vi "Up Down Hall.vi"() -> ()   [LabVIEW 2025]
uses:
  6c21c491-3613-49b9-8739-58848ace7e6b.vi
  9d677228-37d7-4fae-91d8-cc659d765936.vi
  9a2c7101-15d1-4822-83f9-fc476c468639.vi
  af5d74b8-55dd-445e-b05f-4c49f1f30415.vi
panel:
  in  "Save Path":path
  in  "Stop":bool
  in  "Save":bool
  in  "Configuration":T1={"Up file"=path "\\\\myhome\\NHMFLDATA/Data/Cell8daq/Mijkhail Eremets_P20272-E005-PF/October_2025/100825/p154355_100825.tdms", "Down file"=path "\\\\myhome\\NHMFLDATA/Data/Cell8daq/Mijkhail Eremets_P20272-E005-PF/October_2025/100825/p171857_100825.tdms", "Invert X"=TRUE, "Bin data"=enum."Down", "Bin size"=0.1, "Chan Vxy X"="V X1 (Resampled)", "Chan Vxy Y"="V Y1 (Resampled)", "Chan X"="Field (Resampled)", "Group"="p", "Phase"=20.31092436974791, "Delta Phase"=-1.3313253012048292, "Averaging"=0.0, "Output file name"="Hall_250K", "VHall Volts to Ohms"=7.7, "Reference Rhall"=0.0, "Save with zero offset"=TRUE} {"Delta Phase" step=0.05 scale=-180.0..180.0; "Phase" scale=-180.0..180.0}
  out "Hall":T2(graph)
  out "Vxy":T2(graph)
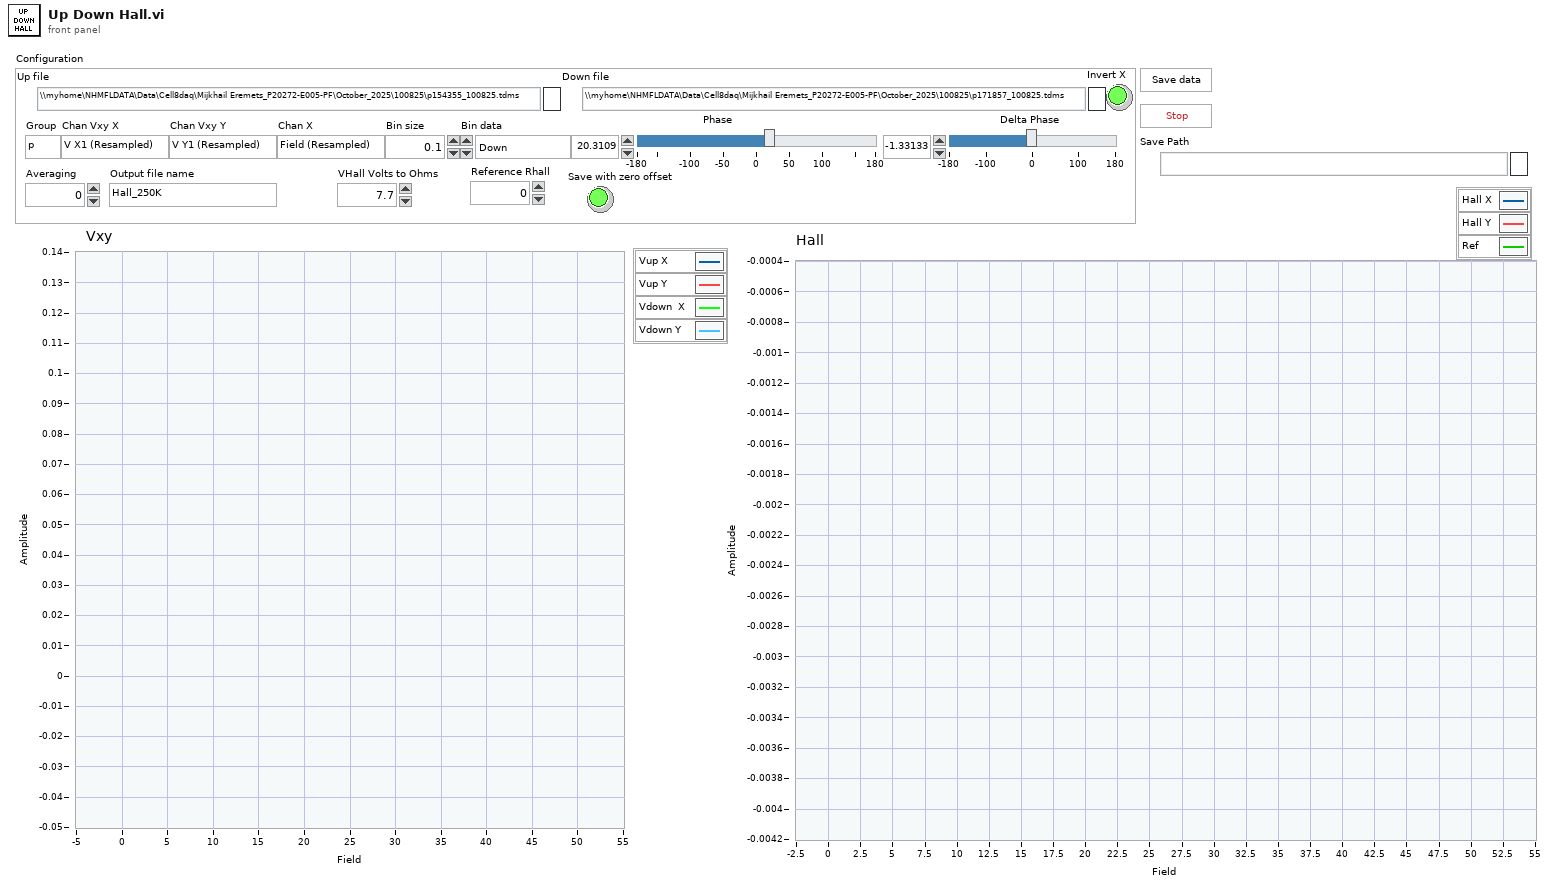
[diagram p1: front panel]
types:
  T1 = cluster{"Up file":path, "Down file":path, "Invert X":bool, "Bin data":enum16{"NONE", "Up", "Down", "Up+Down"}, "Bin size":dbl, "Chan Vxy X":string, "Chan Vxy Y":string, "Chan X":string, "Group":string, "Phase":dbl, "Delta Phase":dbl, "Averaging":dbl, "Output file name":string, "VHall Volts to Ohms":dbl, "Reference Rhall":dbl, "Save with zero offset":bool}
  T2 = cluster{"Binned data up":dbl[], "Binned data up":dbl[]}[]
  T3 = enum16{"open", "open or create", "create or replace", "create", "open (read-only)"}
  T4 = cluster{"Binned data down":dbl[], "Array X out":dbl[]}
  T5 = cluster{"Binned data down":dbl[], "Array Y out":dbl[]}
  T6 = cluster{"Binned data down":dbl[], "Array Y out":dbl[]}[]
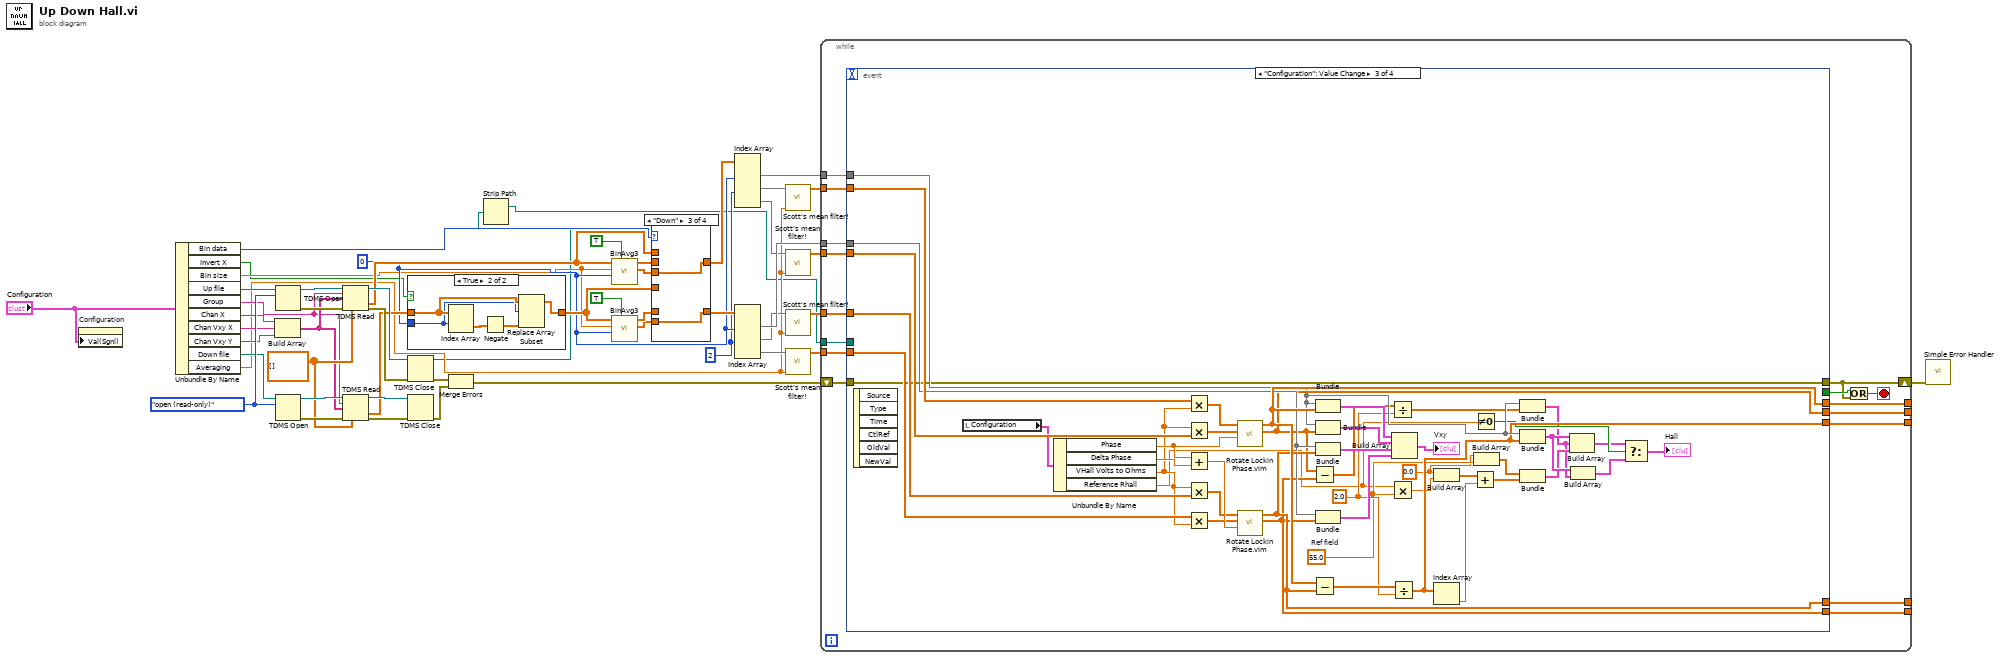
[diagram p0: block diagram]
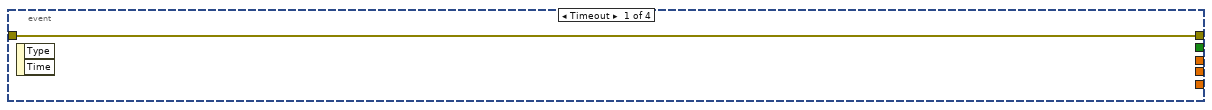
[diagram p3: hidden frame]
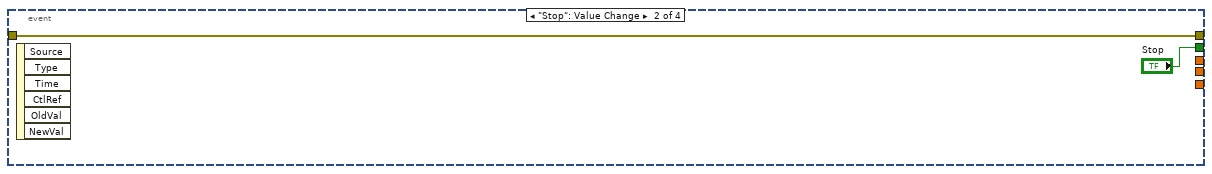
[diagram p4: hidden frame]
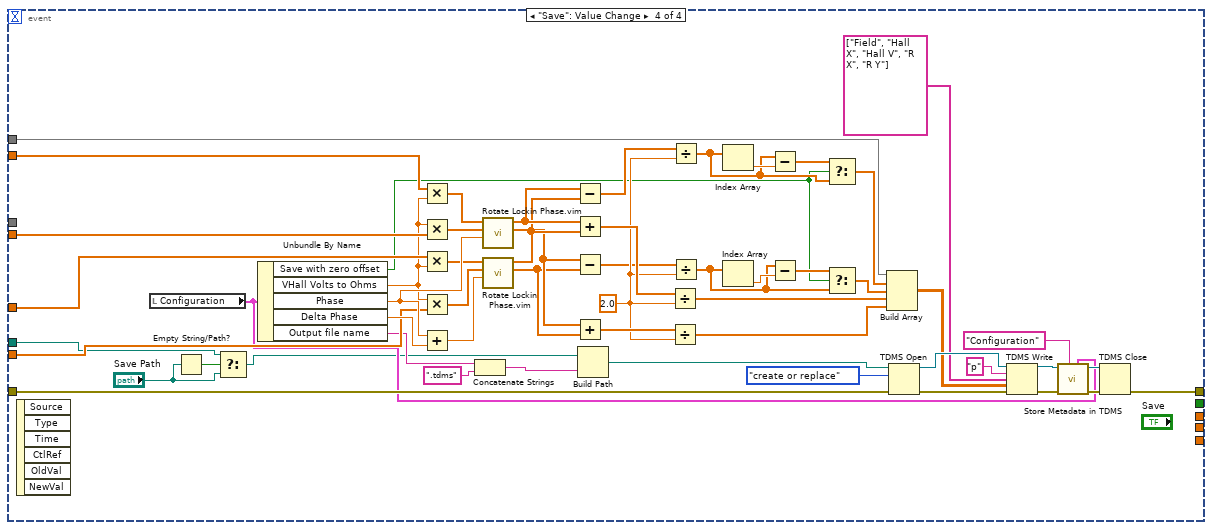
[diagram p5: hidden frame]
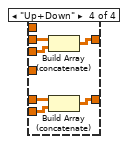
[diagram p8: hidden frame]
diagram:
  w20 = 2 ("index (row)")
  w21 = 0 ("index (row)")
  w42 = dbl[][] []
  w43 = T3."open (read-only)" ("operation (0:open)")
  n1 = property on="Configuration" class="Clust (strict)"("Val(Sgnl)"="Configuration") -> ()  [unwired: 2 in, 2 out]
  n2 = Unbundle By Name("Configuration") -> ("Bin data"=w8:enum16{"NONE", "Up", "Down", "Up+Down"}, "Invert X"=w7:bool, "Bin size"=w11:dbl, "Up file"=w19:path, "Group"=w15:string, "Chan X"=w16:string, "Chan Vxy X"=w18:string, "Chan Vxy Y"=w17:string, "Down file"=w14:path, "Averaging"=w10:dbl)
  n3 = Build Array(w16, w18, w17) -> (w41:string[])
  n4 = TDMS Open(10:w43, 11:w19) -> (0:w50:errorcluster, 3:w51:refnum<k34>)  [unwired: 5 in]
  n5 = TDMS Open(10:w43, 11:w14) -> (0:w45:errorcluster, 3:w44:refnum<k34>)  [unwired: 5 in]
  n6 = TDMS Read(0:w51, 5:w15, 7:w41, 11:w50, 12:w42) -> (4:w48:refnum<k34>, 10:w38:dbl[][], 15:w49:errorcluster)  [unwired: 3 in, 3 out]
  n7 = TDMS Read(0:w44, 5:w15, 7:w41, 11:w45, 12:w42) -> (4:w47:refnum<k34>, 10:w23:dbl[][], 15:w46:errorcluster)  [unwired: 3 in, 3 out]
  n8 = case shown="True" w7 {
    tunnel: w23 -> [w52 w57]
    tunnel: w21 -> [_ w54]
    tunnel: [w52 w53] -> w22
    frame False {
    }
    frame True {
      n9 = Index Array(array=w57, index (row)=w54) -> (element=w56:dbl[])  [unwired: 1 in]
      n10 = Negate(x=w56) -> (-x=w55:dbl[])
      n11 = Replace Array Subset(array=w57, new element=w55, index (row)=w54) -> (w53:dbl[][])  [unwired: 1 in]
    }
  }
  n12 = TDMS Close(8:w49, 11:w48) -> (0:w3:errorcluster, 3:w6:path)
  n13 = TDMS Close(8:w46, 11:w47) -> (0:w4:errorcluster)  [unwired: 1 out]
  n14 = Merge Errors(w3, w4) -> (w2:errorcluster)
  n15 = Strip Path(path=w6) -> (stripped path=w5:path)  [unwired: 1 out]
  n16 = call "BinAvg3.vi"("Extend to 0"=TRUE, "X coumn index"=w21, "Bin size"=w11, "Data in"=w38) -> ("Binned data down"=w36:dbl[][], "Binned data up"=w39:dbl[][])  [unwired: 6 in]
  n17 = call "BinAvg3.vi"("Extend to 0"=TRUE, "X coumn index"=w21, "Bin size"=w11, "Data in"=w22) -> ("Binned data down"=w37:dbl[][], "Binned data up"=w40:dbl[][])  [unwired: 6 in]
  n18 = case shown="\"Down\"" w8 {
    tunnel: w40 -> [_ w61 _ w69]
    tunnel: [w59 w61 w63 w67] -> w29
    tunnel: w39 -> [_ w60 _ w66]
    tunnel: [w58 w60 w62 w64] -> w35
    tunnel: w22 -> [w59 _ _ _]
    tunnel: w38 -> [w58 _ _ _]
    tunnel: w37 -> [_ _ w63 w68]
    tunnel: w36 -> [_ _ w62 w65]
    frame "NONE", Default {
    }
    frame "Up" {
    }
    frame "Down" {
    }
    frame "Up+Down" {
      n19 = Build Array (concatenate)(w66, w65) -> (w64:dbl[][])
      n20 = Build Array (concatenate)(w69, w68) -> (w67:dbl[][])
    }
  }
  n21 = Index Array(array=w35, index (col) #1=w21, index (col) #2=w20) -> (element #1=w34:dbl[], element #2=w25:dbl[], element #3=w24:dbl[])  [unwired: 4 in]
  n22 = Index Array(array=w29, index (col) #1=w21, index (col) #2=w20) -> (element #1=w28:dbl[], element #2=w27:dbl[], element #3=w26:dbl[])  [unwired: 4 in]
  n23 = call "Scott's mean filter!.vi"("window size"=w10, "input"=w25) -> ("output"=w33:dbl[])  [unwired: 9 out]
  n24 = call "Scott's mean filter!.vi"("window size"=w10, "input"=w24) -> ("output"=w32:dbl[])  [unwired: 9 out]
  n25 = call "Scott's mean filter!.vi"("window size"=w10, "input"=w27) -> ("output"=w31:dbl[])  [unwired: 9 out]
  n26 = call "Scott's mean filter!.vi"("window size"=w10, "input"=w26) -> ("output"=w30:dbl[])  [unwired: 9 out]
  n27 = while {
    tunnel: [w78] -> _
    tunnel: [w80] -> _
    tunnel: [w77] -> _
    tunnel: [w81] -> _
    tunnel: [w79] -> _
    tunnel: w30 -> [w82]
    tunnel: w31 -> [w83]
    tunnel: w32 -> [w84]
    tunnel: w33 -> [w85]
    tunnel: w34 -> [w75]
    tunnel: w28 -> [w74]
    tunnel: w5 -> [w73]
    shift-right: [w71] -> w1
    shift-left: w2 -> [w70]
    stop <- w72 stop-if-true
    n28 = event shown="[2] \"Configuration\": Value Change" {
      selector: _ -> [_ _ _ _]
      dyn-events: _ -> [_ _ _ _]
      timeout: _ -> [_ _ _ _]
      tunnel: w85 -> [_ _ w133 w184]
      tunnel: w84 -> [_ _ w132 w183]
      tunnel: w83 -> [_ _ w131 w151]
      tunnel: w82 -> [_ _ w130 w182]
      tunnel: [_ _ w121 _] -> w81
      tunnel: [_ _ w120 _] -> w80
      tunnel: [_ _ w129 _] -> w79
      tunnel: [_ _ w104 _] -> w78
      tunnel: [_ _ w125 _] -> w77
      tunnel: [_ "Stop" _ _] -> w76
      tunnel: w75 -> [_ _ w119 w185]
      tunnel: w74 -> [_ _ w124 _]
      tunnel: w73 -> [_ _ _ w148]
      tunnel: w70 -> [w86 w87 w114 w178]
      tunnel: [w86 w87 w114 w173] -> w71
      event Timeout {
        n29 = event-data() -> ()  [unwired: 3 out]
      }
      event "Stop": Value Change {
        n30 = event-data() -> ()  [unwired: 7 out]
      }
      event "Configuration": Value Change {
        w100 = 0.0 ("element")
        w101 = 55.0  # Ref field
        w105 = 2.0
        n31 = event-data() -> ()  [unwired: 7 out]
        n32 = local read "Configuration"() -> (w117:T1)
        n33 = Unbundle By Name(w117) -> ("Phase"=w116:dbl, "Delta Phase"=w115:dbl, "VHall Volts to Ohms"=w109:dbl, "Reference Rhall"=w90:dbl)
        n34 = Multiply(x=w133, y=w109) -> (x*y=w113:dbl[])
        n35 = Multiply(x=w109, y=w132) -> (x*y=w112:dbl[])
        n36 = Add(x=w116, y=w115) -> (x+y=w118:dbl)
        n37 = Multiply(x=w109, y=w131) -> (x*y=w111:dbl[])
        n38 = Multiply(x=w130, y=w109) -> (x*y=w110:dbl[])
        n39 = call "Rotate Lockin Phase.vim"("Phase"=w116, "Array Y in"=w112, "Array X in"=w113) -> ("Array Y out"=w121:dbl[], "Array X out"=w129:dbl[])  [unwired: 7 in]
        n40 = call "Rotate Lockin Phase.vim"("Phase"=w118, "Array Y in"=w110, "Array X in"=w111) -> ("Array Y out"=w120:dbl[], "Array X out"=w125:dbl[])  [unwired: 7 in]
        n41 = Subtract(x=w121, y=w120) -> (x-y=w107:dbl[])
        n42 = Subtract(x=w129, y=w125) -> (x-y=w106:dbl[])
        n43 = Bundle("Binned data down"=w119, "Array X out"=w129) -> (w128:T4)  [unwired: 1 in]
        n44 = Bundle("Binned data down"=w119, "Array Y out"=w121) -> (w127:T5)  [unwired: 1 in]
        n45 = Bundle("Binned data down"=w124, "Array X out"=w125) -> (w122:T4)  [unwired: 1 in]
        n46 = Bundle("Binned data down"=w124, "Array Y out"=w120) -> (w123:T5)  [unwired: 1 in]
        n47 = Divide(x=w107, y=w105) -> (x/y=w108:dbl[])
        n48 = Multiply(x=w90, y=w101) -> (x*y=w99:dbl)
        n49 = Divide(x=w106, y=w105) -> (x/y=w104:dbl[])
        n50 = Build Array(w128, w127, w122, w123) -> (→"Vxy":T6)
        n51 = Build Array(w100, w99) -> (w97:dbl[])
        n52 = Index Array(array=w104) -> (element=w102:dbl)  [unwired: 1 in]
        n53 = Add(x=w97, y=w102) -> (x+y=w103:dbl[])
        n54 = Not Equal To 0?(x=w90) -> (x != 0?=w96:bool)
        n55 = Build Array(w100, w101) -> (w98:dbl[])
        n56 = Bundle("Binned data down"=w119, w108) -> (w89:cluster{"Binned data down":dbl[], dbl[]})  [unwired: 1 in]
        n57 = Bundle("Binned data down"=w119, w104) -> (w93:cluster{"Binned data down":dbl[], dbl[]})  [unwired: 1 in]
        n58 = Bundle(w98, w103) -> (w92:cluster{dbl[], dbl[]})  [unwired: 1 in]
        n59 = Build Array(w93, w89, w92) -> (w95:cluster{"Binned data down":dbl[], dbl[]}[])
        n60 = Build Array(w93, w89) -> (w91:cluster{"Binned data down":dbl[], dbl[]}[])
        n61 = Select(t=w95, s=w96, f=w91) -> (s? t:f=→"Hall":cluster{"Binned data down":dbl[], dbl[]}[])
      }
      event "Save": Value Change {
        w145 = 2.0
        n62 = event-data() -> ()  [unwired: 7 out]
        n63 = local read "Configuration"() -> (w165:T1)
        n64 = Empty String/Path?(string/path="Save Path") -> (empty?=w149:bool)
        n65 = Select(t=w148, s=w149, f="Save Path") -> (s? t:f=w146:path)
        n66 = Unbundle By Name(w165) -> ("Save with zero offset"=w135:bool, "VHall Volts to Ohms"=w150:dbl, "Phase"=w187:dbl, "Delta Phase"=w186:dbl, "Output file name"=w181:string)
        n67 = Multiply(x=w184, y=w150) -> (x*y=w152:dbl[])
        n68 = Multiply(x=w150, y=w183) -> (x*y=w153:dbl[])
        n69 = Multiply(x=w151, y=w150) -> (x*y=w154:dbl[])
        n70 = Multiply(x=w150, y=w182) -> (x*y=w155:dbl[])
        n71 = Add(x=w187, y=w186) -> (x+y=w188:dbl)
        n72 = Concatenate Strings(w181, ".tdms") -> (w179:string)
        n73 = call "Rotate Lockin Phase.vim"("Phase"=w187, "Array Y in"=w153, "Array X in"=w152) -> ("Array Y out"=w161:dbl[], "Array X out"=w163:dbl[])  [unwired: 7 in]
        n74 = call "Rotate Lockin Phase.vim"("Phase"=w188, "Array Y in"=w155, "Array X in"=w154) -> ("Array Y out"=w160:dbl[], "Array X out"=w162:dbl[])  [unwired: 7 in]
        n75 = Subtract(x=w163, y=w162) -> (x-y=w144:dbl[])
        n76 = Add(x=w163, y=w162) -> (x+y=w159:dbl[])
        n77 = Subtract(x=w161, y=w160) -> (x-y=w143:dbl[])
        n78 = Add(x=w161, y=w160) -> (x+y=w158:dbl[])
        n79 = Build Path(base path=w146, name or relative path=w179) -> (appended path=w177:path)
        n80 = Divide(x=w159, y=w145) -> (x/y=w157:dbl[])
        n81 = Divide(x=w158, y=w145) -> (x/y=w156:dbl[])
        n82 = Divide(x=w144, y=w145) -> (x/y=w140:dbl[])
        n83 = Divide(x=w143, y=w145) -> (x/y=w136:dbl[])
        n84 = Index Array(array=w140) -> (element=w142:dbl)  [unwired: 1 in]
        n85 = Index Array(array=w136) -> (element=w137:dbl)  [unwired: 1 in]
        n86 = Subtract(x=w140, y=w142) -> (x-y=w141:dbl[])
        n87 = Subtract(x=w136, y=w137) -> (x-y=w138:dbl[])
        n88 = Select(t=w141, s=w135, f=w140) -> (s? t:f=w139:dbl[])
        n89 = Select(t=w138, s=w135, f=w136) -> (s? t:f=w134:dbl[])
        n90 = Build Array(w185, w139, w134, w157, w156) -> (w170:dbl[][])
        n91 = TDMS Open(8:w178, 10:T3."create or replace" ("operation (0:open)"), 11:w177) -> (0:w175:errorcluster, 3:w174:refnum<k34>)  [unwired: 4 in]
        n92 = TDMS Write(0:w174, 5:"p" ("group name in (Untitled)"), 7:string[] ["Field", "Hall X", "Hall V", "R X", "R Y"] ("channel name(s) in (Untitled)"), 9:w170, 11:w175) -> (4:w169:refnum<k34>, 15:w166:errorcluster)  [unwired: 1 in, 2 out]
        n93 = call "Store Metadata in TDMS.vi"("Value"=w165, "name"="Configuration", "Error In"=w166, "tdms file"=w169) -> ("Error Out"=w167:errorcluster, "tdms file out"=w168:refnum<k34>)  [unwired: 3 in, 3 out]
        n94 = TDMS Close(8:w167, 11:w168) -> (0:w173:errorcluster)  [unwired: 1 out]
      }
    }
    n95 = Or(x=w76, y=w71) -> (x .or. y?=w72:bool)
  }
  n96 = call <vilib>:"Simple Error Handler.vi"("error in (no error)"=w1) -> ()  [unwired: 4 in, 5 out]
